vi "Returning A Value Array Of Integers.vi"(8 "error in (no error)":errorcluster, 11 "length":i32) -> (0 "error out":errorcluster, 3 "function return":i32)   [LabVIEW 2009, in "LabVIEWWrapper_PassingDataSampleDLL.lvlib"]
doc: "int* ReturningAValue_ArrayOfIntegers (int length);"
uses:
  LabVIEWWrapper_PassingDataSampleDLL.lvlib
  PassingDataSampleDLL.dll
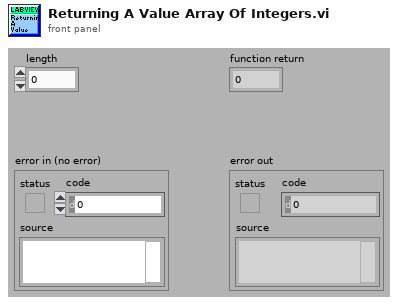
[diagram p1: front panel]
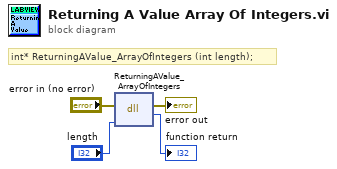
[diagram p0: block diagram]
diagram:
  # "int* ReturningAValue_ArrayOfIntegers (int length);"
  n1 = dll-call lib="C:/My Dropbox/Systems Engineering Application/SDK/C Integration/LabVIEWWrapper/PassingDataSampleDLL.*" fn="ReturningAValue_ArrayOfIntegers"(error in="error in (no error)", "length"="length") -> (error out=→"error out":errorcluster, →"function return":i32)  [unwired: 3 in, 1 out]
